vi "Write settings.vi"(8 "error in (no error)":errorcluster, 10 "settings":T1={"VISA resource name"="", "baud rate (9600)"=9600, "timeout (10sec)"=10000, "termination char\n(0xA = '\\n' = LF) "=10, "Enable Termination\nChar (T)"=TRUE, "data bits (8)"=8, "parity (0:none)"=enum."None"} {"baud rate (9600)" items=["75"=75, "110"=110, "134"=134, "150"=150, "300"=300, "600"=600, "1200"=1200, "1800"=1800, "2400"=2400, "4800"=4800, "7200"=7200, "9600"=9600, "14400"=14400, "19200"=19200, "28800"=28800, "38400"=38400, "56000"=56000, "57600"=57600, "115200"=115200, "128000"=128000, "230400"=230400]}, 11 "HP-S-Serial in":refnum<class "HP-S-Serial.lvclass">) -> (0 "error out":errorcluster, 3 "HP-S-Serial out":refnum<class "HP-S-Serial.lvclass">)   [LabVIEW 2020, in "HP-S-Serial.lvclass"]
uses:
  HP-S-Serial.lvclass
  HP-S-settings.ctl
  HP-S-baudrate.ctl
  HP-S-Serial.lvclass/HP-S-Serial.ctl
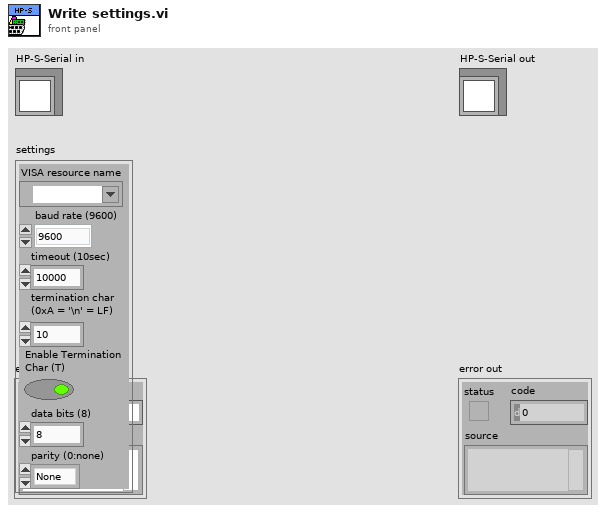
[diagram p1: front panel]
types:
  T1 = typedef "HP-S-Serial.lvclass/HP-S-settings.ctl" = cluster{"VISA resource name":refnum<visa-resource-name>, "baud rate (9600)":T2, "timeout (10sec)":u32, "termination char\n(0xA = '\\n' = LF) ":u8, "Enable Termination\nChar (T)":bool, "data bits (8)":u16, "parity (0:none)":enum16{"None", "Odd", "Even", "Mark", "Space"}}
  T2 = typedef "HP-S-Serial.lvclass/HP-S-baudrate.ctl" = u32
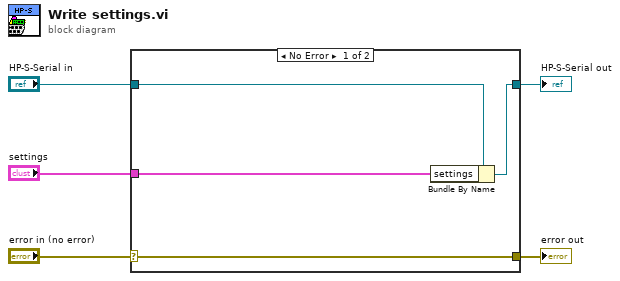
[diagram p0: block diagram]
diagram:
  n1 = case shown="No Error" "error in (no error)" {
    selector: "error in (no error)" -> [w9 w10]
    tunnel: [w9 w10] -> w4
    tunnel: [w7 w11] -> w2
    tunnel: "HP-S-Serial in" -> [w8 w11]
    tunnel: "settings" -> [w6 _]
    frame No Error {
      n2 = Bundle By Name(cluster=w8, "settings"=w6) -> (w7:refnum<class "HP-S-Serial.lvclass">)
    }
    frame Error {
    }
  }
  "error out" <- w4
  "HP-S-Serial out" <- w2
